vi "Bench n Squat.vi"() -> ()   [LabVIEW 2009]
uses:
  <vilib>/Utility/file.llb/Read From Spreadsheet File (string).vi
  <vilib>/Utility/file.llb/Write To Spreadsheet File (string).vi
panel:
  in  "Delete last":bool
  in  "TODAYS DATA":string[](array[string])=["REPS COMPLETED", "Squat (kg)", "Bench (kg)"]
  out "output data from session":string[][](array[string])
  in  "STOP session":bool
  out "transposed array":string[][](array[string])
  out "player DATA":string[][](array[string])
  out "data to save":string[][](array[string])
  out "new data":string[](array[string])
  in  "START":bool
  in  "DATE":string
  out "Input file data":string[][](array[string])
  in  "PLAYER NAME":string(combo)
  in  "SQUAT":bool
  in  "BENCH":bool
  in  "LOAD (kg)":string
  in  "REPS COMPLETED":string(combo)
  in  "Data file":path caption="DATA FILE"
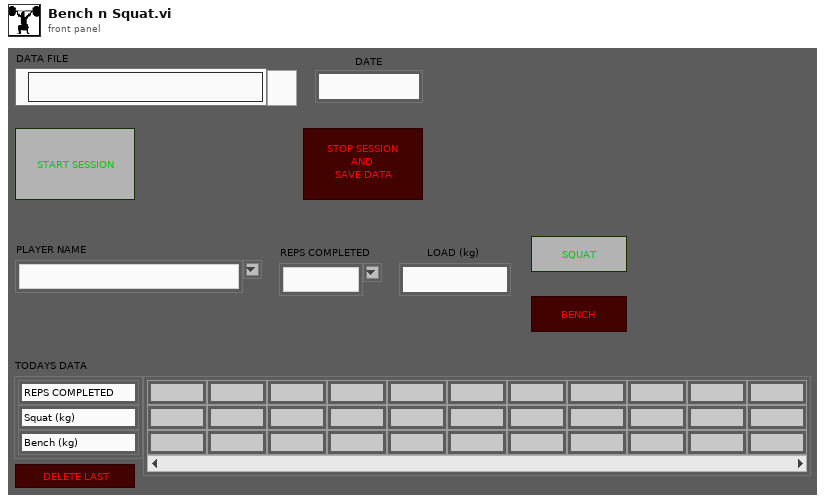
[diagram p1: front panel]
types:
  T1 = enum8{"Enabled", "Disabled", "Disabled and Grayed Out"}
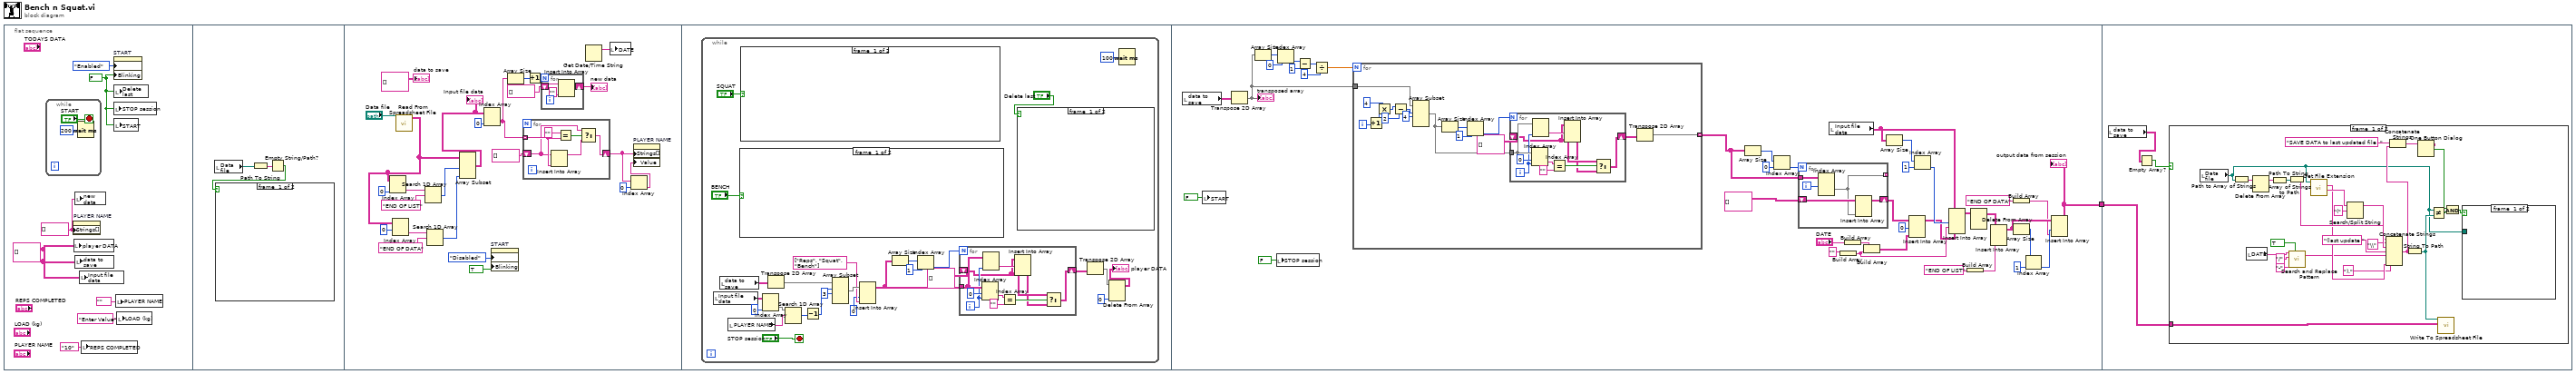
[diagram p0: block diagram]
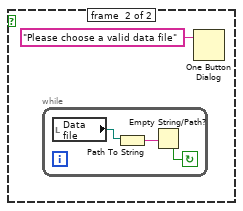
[diagram p2: hidden frame]
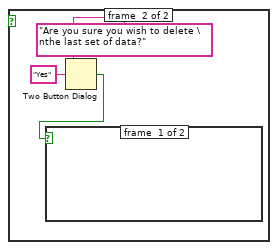
[diagram p3: hidden frame]
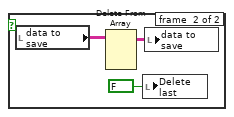
[diagram p4: hidden frame]
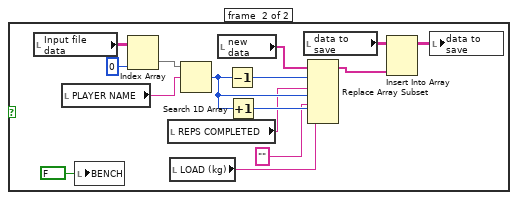
[diagram p5: hidden frame]
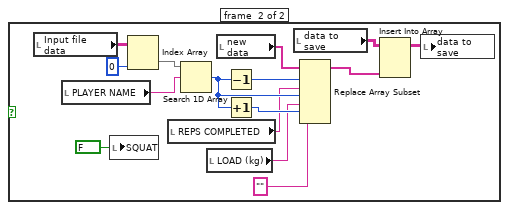
[diagram p6: hidden frame]
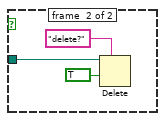
[diagram p7: hidden frame]
diagram:
  n1 = flat-sequence {
    tunnel: [w126] -> w1
    tunnel: w1 -> [w195]
    frame #0 {
      w2 = string[][] [] ("data to save")
      w3 = string[] [] ("Strings []")
      w5 = FALSE ("Blinking")
      n2 = while {
        stop <- "START" stop-if-true
        n3 = Wait (ms)(milliseconds to wait=u32 200) -> ()  [unwired: 1 out]
      }
      n4 = property on="PLAYER NAME" class="CmbBox"("Strings[]"=w3) -> ()  [unwired: 2 in, 2 out]
      n5 = local write "player DATA"(w2) -> ()
      n6 = local write "new data"(w3) -> ()
      n7 = local write "data to save"(w2) -> ()
      n8 = local write "Input file data"(w2) -> ()
      n9 = local write "REPS COMPLETED"("10" ("REPS Completed")) -> ()
      n10 = property on="START" class="Bool (strict)"("DisabledEnum"=T1."Enabled" ("Disabled"), "Blinking"=w5) -> ()  [unwired: 2 in, 2 out]
      n11 = local write "STOP session"(w5) -> ()
      n12 = local write "Delete last"(w5) -> ()
      n13 = local write "START"(w5) -> ()
      n14 = local write "PLAYER NAME"("" ("PLAYER NAME")) -> ()
      n15 = local write "LOAD (kg)"("Enter Value" ("Load (kg)")) -> ()
    }
    frame #1 {
      n16 = local read "Data file"() -> (w13:path)
      n17 = Path To String(path=w13) -> (string=w12:string)
      n18 = Empty String/Path?(string/path=w12) -> (empty?=w11:bool)
      n19 = case shown="True" w11 {
        frame #0 {
        }
        frame #1 {
          n20 = while {
            stop <- w16 continue-if-true
            n21 = local read "Data file"() -> (w15:path)
            n22 = Path To String(path=w15) -> (string=w17:string)
            n23 = Empty String/Path?(string/path=w17) -> (empty?=w16:bool)
          }
          n24 = One Button Dialog(message="Please choose a valid data file") -> ()  [unwired: 1 in, 1 out]
        }
      }
    }
    frame #2 {
      n25 = call-poly <vilib>:"Read From Spreadsheet File.vi"("file path (dialog if empty)"="Data file") -> ("all rows"=w20:string[][])  [unwired: 6 in, 4 out]
      n26 = Index Array(array=w20, index (col)=0 ("disabled index (col)")) -> (element=w33:string[])  [unwired: 1 in]
      n27 = Index Array(array=w20, index (row)=0 ("disabled index (col)")) -> (element=w21:string[])  [unwired: 1 in]
      n28 = Search 1D Array(1D array=w33, element="END OF LIST") -> (index of element=w31:i32)  [unwired: 1 in]
      n29 = Search 1D Array(1D array=w21, element="END OF DATA") -> (index of element=w19:i32)  [unwired: 1 in]
      n30 = Array Subset(array=w20, length (row)=w31, length (col)=w19) -> (w30:string[][])  [unwired: 2 in]
      "Input file data" <- w30
      n31 = Index Array(array=w30, index (col)=0 ("disabled index (col)")) -> (element=w38:string[])  [unwired: 1 in]
      n32 = property on="START" class="Bool (strict)"("DisabledEnum"=T1."Disabled" ("Disabled"), "Blinking"=TRUE) -> ()  [unwired: 2 in, 2 out]
      n33 = Array Size(array=w38) -> (size(s)=w29:i32)
      n34 = for {
        tunnel: w38 -> [w51] mode=indexing
        shift-right: [w46] -> w25
        shift-left: string[] [] ("subarray") -> [w48]
        n35 = Insert Into Array(array=w48, new element=w51) -> (w47:string[])  [unwired: 1 in]
        n36 = Equal?(x="", y=w51) -> (x = y?=w49:bool)
        n37 = Select(t=w48, s=w49, f=w47) -> (s? t:f=w46:string[])
      }
      n38 = Increment(x=w29) -> (x+1=w28:i32)
      n39 = for {
        N: w28 -> [_]
        shift-right: [w44] -> w36
        shift-left: string[] [] -> [w43]
        n40 = Insert Into Array(array=w43, new element="" ("String")) -> (w44:string[])  [unwired: 1 in]
      }
      "new data" <- w36
      n41 = Get Date/Time String() -> (date string=w39:string)  [unwired: 3 in, 1 out]
      n42 = local write "DATE"(w39) -> ()
      n43 = Index Array(array=w25, index=0) -> (element=w23:string)
      n44 = property on="PLAYER NAME" class="CmbBox"("Strings[]"=w25, "Value"=w23) -> ()  [unwired: 2 in, 2 out]
      "data to save" <- string[][] [] ("data to save")
    }
    frame #3 {
      n45 = while {
        stop <- "STOP session" stop-if-true
        n46 = local read "Input file data"() -> (w70:string[][])
        n47 = local read "data to save"() -> (w74:string[][])
        n48 = local read "PLAYER NAME"() -> (w73:string)
        n49 = case shown="True" "BENCH" {
          frame #0 {
          }
          frame #1 {
            n50 = local read "Input file data"() -> (w108:string[][])
            n51 = local read "PLAYER NAME"() -> (w105:string)
            n52 = local write "BENCH"(FALSE ("SQUAT")) -> ()
            n53 = Index Array(array=w108, index (col)=0 ("disabled index (col)")) -> (element=w106:string[])  [unwired: 1 in]
            n54 = local read "REPS COMPLETED"() -> (w100:string)
            n55 = local read "LOAD (kg)"() -> (w97:string)
            n56 = Search 1D Array(1D array=w106, element=w105) -> (index of element=w101:i32)  [unwired: 1 in]
            n57 = local read "new data"() -> (w104:string[])
            n58 = Decrement(x=w101) -> (x-1=w102:i32)
            n59 = Increment(x=w101) -> (x+1=w103:i32)
            n60 = local read "data to save"() -> (w96:string[][])
            n61 = Replace Array Subset(array=w104, new element #1=w100, index #1=w102, new element #2="" ("String"), index #2=w101, new element #3=w97, index #3=w103) -> (w95:string[])
            n62 = Insert Into Array(array=w96, new element=w95) -> (w94:string[][])  [unwired: 2 in]
            n63 = local write "data to save"(w94) -> ()
          }
        }
        n64 = case shown="True" "SQUAT" {
          frame #0 {
          }
          frame #1 {
            n65 = local read "Input file data"() -> (w123:string[][])
            n66 = local read "PLAYER NAME"() -> (w120:string)
            n67 = local write "SQUAT"(FALSE ("SQUAT")) -> ()
            n68 = Index Array(array=w123, index (col)=0 ("disabled index (col)")) -> (element=w121:string[])  [unwired: 1 in]
            n69 = local read "REPS COMPLETED"() -> (w115:string)
            n70 = Search 1D Array(1D array=w121, element=w120) -> (index of element=w116:i32)  [unwired: 1 in]
            n71 = local read "LOAD (kg)"() -> (w114:string)
            n72 = local read "new data"() -> (w119:string[])
            n73 = Decrement(x=w116) -> (x-1=w117:i32)
            n74 = Increment(x=w116) -> (x+1=w118:i32)
            n75 = local read "data to save"() -> (w111:string[][])
            n76 = Replace Array Subset(array=w119, new element #1=w115, index #1=w117, new element #2=w114, index #2=w116, new element #3="" ("String"), index #3=w118) -> (w109:string[])
            n77 = Insert Into Array(array=w111, new element=w109) -> (w110:string[][])  [unwired: 2 in]
            n78 = local write "data to save"(w110) -> ()
          }
        }
        n79 = Index Array(array=w70, index (col)=0 ("disabled index (col)")) -> (element=w72:string[])  [unwired: 1 in]
        n80 = Transpose 2D Array(2D array=w74) -> (transposed array=w69:string[][])
        n81 = Search 1D Array(1D array=w72, element=w73) -> (index of element=w68:i32)  [unwired: 1 in]
        n82 = Decrement(x=w68) -> (x-1=w67:i32)
        n83 = Array Subset(array=w69, index (row)=w67, length (row)=3 ("length")) -> (w65:string[][])  [unwired: 2 in]
        n84 = Insert Into Array(array=w65, index (col)=0 ("disabled index (col)"), new element=string[] ["Reps", "Squat", "Bench"]) -> (w62:string[][])  [unwired: 1 in]
        n85 = Array Size(array=w62) -> (size(s)=w61:i32[])
        n86 = Index Array(array=w61, index=1) -> (element=w59:i32)
        n87 = for {
          N: w59 -> [_]
          tunnel: w62 -> [w90]
          shift-right: [w86] -> w57
          shift-left: string[][] [] -> [w85]
          i -> [w89]
          n88 = Index Array(array=w90, index (row)=0, index (col)=w89) -> (element=w92:string)
          n89 = Index Array(array=w90, index (col)=w89) -> (element=w88:string[])  [unwired: 1 in]
          n90 = Equal?(x=w92, y="") -> (x = y?=w87:bool)
          n91 = Insert Into Array(array=w85, new element=w88) -> (w84:string[][])  [unwired: 2 in]
          n92 = Select(t=w85, s=w87, f=w84) -> (s? t:f=w86:string[][])
        }
        n93 = case shown="True" "Delete last" {
          frame #0 {
          }
          frame #1 {
            n94 = Two Button Dialog(message="Are you sure you wish to delete \nthe last set of data?", 2:"Yes" ("T button name (\"OK\")")) -> (T button?=w79:bool)  [unwired: 1 in]
            n95 = case shown="True" w79 {
              frame #0 {
              }
              frame #1 {
                n96 = local read "data to save"() -> (w83:string[][])
                n97 = Delete From Array(array=w83) -> (array with subset deleted=w82:string[][])  [unwired: 3 in, 1 out]
                n98 = local write "Delete last"(FALSE ("Delete last")) -> ()
                n99 = local write "data to save"(w82) -> ()
              }
            }
          }
        }
        n100 = Transpose 2D Array(2D array=w57) -> (transposed array=w55:string[][])
        n101 = Delete From Array(array=w55, index (col)=0 ("disabled index (col)")) -> (array with subset deleted=→"player DATA":string[][])  [unwired: 2 in, 1 out]
        n102 = Wait (ms)(milliseconds to wait=u32 100) -> ()  [unwired: 1 out]
      }
    }
    frame #4 {
      n103 = local read "data to save"() -> (w162:string[][])
      n104 = local write "START"(FALSE ("START")) -> ()
      n105 = Transpose 2D Array(2D array=w162) -> (transposed array=w155:string[][])
      "transposed array" <- w155
      n106 = Array Size(array=w155) -> (size(s)=w161:i32[])
      n107 = local write "STOP session"(FALSE ("STOP session")) -> ()
      n108 = Index Array(array=w161, index=0) -> (element=w159:i32)
      n109 = Subtract(x=w159, y=1) -> (x-y=w157:i32)
      n110 = Divide(x=w157, y=4) -> (x/y=w149:dbl)
      n111 = for {
        N: w149 -> [_]
        tunnel: w155 -> [w179]
        tunnel: [w168] -> w141 mode=indexing
        i -> [w172]
        n112 = Increment(x=w172) -> (x+1=w171:i32)
        n113 = Multiply(x=4, y=w171) -> (x*y=w170:i32)
        n114 = Subtract(x=w170, y=2) -> (x-y=w180:i32)
        n115 = Array Subset(array=w179, index (row)=w180, length (row)=4 ("length")) -> (w173:string[][])  [unwired: 2 in]
        n116 = Array Size(array=w173) -> (size(s)=w178:i32[])
        n117 = Index Array(array=w178, index=1) -> (element=w176:i32)
        n118 = for {
          N: w176 -> [_]
          tunnel: w173 -> [w189]
          shift-right: [w185] -> w174
          shift-left: string[][] [] -> [w184]
          i -> [w188]
          n119 = Index Array(array=w189, index (row)=0, index (col)=w188) -> (element=w191:string)
          n120 = Index Array(array=w189, index (col)=w188) -> (element=w187:string[])  [unwired: 1 in]
          n121 = Equal?(x=w191, y="") -> (x = y?=w186:bool)
          n122 = Insert Into Array(array=w184, new element=w187) -> (w183:string[][])  [unwired: 2 in]
          n123 = Select(t=w184, s=w186, f=w183) -> (s? t:f=w185:string[][])
        }
        n124 = Transpose 2D Array(2D array=w174) -> (transposed array=w168:string[][])
      }
      n125 = Array Size(array=w141) -> (size(s)=w154:i32[])
      n126 = Index Array(array=w154, index=0) -> (element=w152:i32)
      n127 = for {
        N: w152 -> [_]
        tunnel: w141 -> [w167]
        shift-right: [w164] -> w148
        shift-left: string[][] [] ("Array") -> [w165]
        tunnel: [w163] -> _ mode=indexing
        i -> [w166]
        n128 = Index Array(array=w167, index (dim 0)=w166) -> (element=w163:string[][])  [unwired: 2 in]
        n129 = Insert Into Array(array=w165, new element=w163) -> (w164:string[][])  [unwired: 2 in]
      }
      n130 = local read "Input file data"() -> (w142:string[][])
      n131 = Build Array("" ("element")) -> (w135:string[])
      n132 = Build Array("DATE") -> (w144:string[])
      n133 = Build Array(w144, w135) -> (w143:string[][])
      n134 = Array Size(array=w142) -> (size(s)=w139:i32[])
      n135 = Insert Into Array(array=w148, index (row)=0, new element=w143) -> (w136:string[][])  [unwired: 1 in]
      n136 = Index Array(array=w139, index=1) -> (element=w138:i32)
      n137 = Insert Into Array(array=w142, index (col)=w138, new element #1=w135, new element #2=w136) -> (w125:string[][])  [unwired: 1 in]
      n138 = Build Array("END OF LIST" ("element")) -> (w130:string[])
      n139 = Delete From Array(array=w125) -> (array with subset deleted=w124:string[][])  [unwired: 3 in, 1 out]
      n140 = Insert Into Array(array=w124, new element=w130) -> (w129:string[][])  [unwired: 2 in]
      n141 = Build Array("END OF DATA" ("element")) -> (w127:string[])
      n142 = Array Size(array=w129) -> (size(s)=w132:i32[])
      n143 = Index Array(array=w132, index=1) -> (element=w131:i32)
      n144 = Insert Into Array(array=w129, index (col)=w131, new element=w127) -> (w126:string[][])  [unwired: 1 in]
      "output data from session" <- w126
    }
    frame #5 {
      n145 = local read "data to save"() -> (w194:string[][])
      n146 = Empty Array?(array=w194) -> (empty?=w193:bool)
      n147 = case shown="False" w193 {
        tunnel: w195 -> [w220 _]
        frame #0 {
          n148 = local read "Data file"() -> (w199:path)
          n149 = Path to Array of Strings(0:w199) -> (2:w212:string[])  [unwired: 1 out]
          n150 = local read "DATE"() -> (w205:string)
          n151 = Delete From Array(array=w212) -> (array with subset deleted=w213:string[])  [unwired: 2 in, 1 out]
          n152 = Array of Strings to Path(0:w213) -> (2:w214:path)  [unwired: 1 in]
          n153 = Path To String(path=w214) -> (string=w216:string)
          n154 = call <vilib>:"Search and Replace Pattern.vi"("string"=w205, "regular expression (\"\")"="/" ("regular expression (\"\")"), "replace string (\"\")"="-" ("replace string (\"\")"), "replace all? (F)"=TRUE) -> ("result string"=w204:string)  [unwired: 1 in, 1 out]
          n155 = call <vilib>:"Get File Extension.vi"("file"=w199) -> ("filename without extension"=w218:string, "lowercase file extension"=w211:string)  [unwired: 7 in, 2 out]
          n156 = Search/Split String(string=w218, search string/char (-)="(") -> (substring before match=w219:string)  [unwired: 1 in, 2 out]
          n157 = Concatenate Strings(w216, "\\" ("string"), w219, "(last update " ("string"), w204, ")." ("string"), w211) -> (w202:string)
          n158 = Concatenate Strings("SAVE DATA to last updated file  " ("message"), w202) -> (w201:string)
          n159 = String To Path(string=w202) -> (path=w200:path)
          n160 = One Button Dialog(message=w201) -> (true=w196:bool)  [unwired: 1 in]
          n161 = Not Equal?(x=w199, y=w200) -> (x != y?=w198:bool)
          n162 = call-poly <vilib>:"Write To Spreadsheet File.vi"("2D data"=w220, "file path (dialog if empty)"=w200) -> ()  [unwired: 6 in, 1 out]
          n163 = And(x=w196, y=w198) -> (x .and. y?=w197:bool)
          n164 = case shown="True" w197 {
            tunnel: w199 -> [_ w223]
            frame #0 {
            }
            frame #1 {
              n165 = Delete(prompt (Delete)="delete?", path (use dialog)=w223, confirm (F)=TRUE) -> ()  [unwired: 2 in, 3 out]
            }
          }
        }
        frame #1 {
        }
      }
    }
  }
